vi "836_SetCameraConfiguration.vi"(6 "Vision Fix":bool, 8 "error in (no error)":errorcluster, 9 "Camera Controls":T1, 10 "Initialize":bool, 11 "CameraDevRef":T3={"Camera Address"="USB 0", "CameraStatus"={"status"=FALSE, "code"=0, "source"=""}}) -> (0 "error out":errorcluster, 1 "VideoMode":T2=78 items=["640 x 480 YUY 2 30.00 fps", "640 x 480 YUY 2 20.00 fps", "640 x 480 YUY 2 15.00 fps", "640 x 480 YUY 2 10.00 fps", "640 x 480 YUY 2 7.50 fps", "1280 x 720 YUY 2 10.00 fps", "1280 x 720 YUY 2 7.50 fps", "960 x 544 YUY 2 15.00 fps", "960 x 544 YUY 2 10.00 fps", "960 x 544 YUY 2 7.50 fps", "800 x 448 YUY 2 20.00 fps", "800 x 448 YUY 2 15.00 fps", "800 x 448 YUY 2 10.00 fps", "800 x 448 YUY 2 7.50 fps", "640 x 360 YUY 2 30.00 fps", "640 x 360 YUY 2 20.00 fps", "640 x 360 YUY 2 15.00 fps", "640 x 360 YUY 2 10.00 fps", "640 x 360 YUY 2 7.50 fps", "424 x 240 YUY 2 30.00 fps", "424 x 240 YUY 2 20.00 fps", "424 x 240 YUY 2 15.00 fps", "424 x 240 YUY 2 10.00 fps", "424 x 240 YUY 2 7.50 fps", "352 x 288 YUY 2 30.00 fps", "352 x 288 YUY 2 20.00 fps", "352 x 288 YUY 2 15.00 fps", "352 x 288 YUY 2 10.00 fps", "352 x 288 YUY 2 7.50 fps", "320 x 240 YUY 2 30.00 fps", "320 x 240 YUY 2 20.00 fps", "320 x 240 YUY 2 15.00 fps", "320 x 240 YUY 2 10.00 fps", "320 x 240 YUY 2 7.50 fps", "800 x 600 YUY 2 15.00 fps", "800 x 600 YUY 2 10.00 fps", "800 x 600 YUY 2 7.50 fps", "176 x 144 YUY 2 30.00 fps", "176 x 144 YUY 2 20.00 fps", "176 x 144 YUY 2 15.00 fps", "176 x 144 YUY 2 10.00 fps", "176 x 144 YUY 2 7.50 fps", "160 x 120 YUY 2 30.00 fps", "160 x 120 YUY 2 20.00 fps", "160 x 120 YUY 2 15.00 fps", "160 x 120 YUY 2 10.00 fps", "160 x 120 YUY 2 7.50 fps", "1280 x 800 YUY 2 10.00 fps", "640 x 480 JPEG 30.00 fps", "640 x 480 JPEG 20.00 fps", "640 x 480 JPEG 15.00 fps", "640 x 480 JPEG 10.00 fps", "640 x 480 JPEG 7.50 fps", "1280 x 720 JPEG 30.00 fps", "1280 x 720 JPEG 20.00 fps", "1280 x 720 JPEG 15.00 fps", "1280 x 720 JPEG 10.00 fps", "1280 x 720 JPEG 7.50 fps", "960 x 544 JPEG 30.00 fps", "960 x 544 JPEG 20.00 fps", "960 x 544 JPEG 15.00 fps", "960 x 544 JPEG 10.00 fps", "960 x 544 JPEG 7.50 fps", "800 x 448 JPEG 30.00 fps", "800 x 448 JPEG 20.00 fps", "800 x 448 JPEG 15.00 fps", "800 x 448 JPEG 10.00 fps", "800 x 448 JPEG 7.50 fps", "640 x 360 JPEG 30.00 fps", "640 x 360 JPEG 20.00 fps", "640 x 360 JPEG 15.00 fps", "640 x 360 JPEG 10.00 fps", "640 x 360 JPEG 7.50 fps", "800 x 600 JPEG 30.00 fps", "800 x 600 JPEG 20.00 fps", "800 x 600 JPEG 15.00 fps", "800 x 600 JPEG 10.00 fps", "800 x 600 JPEG 7.50 fps", "416 x 240 JPEG 30.00 fps", "416 x 240 JPEG 20.00 fps", "416 x 240 JPEG 15.00 fps", "416 x 240 JPEG 10.00 fps", "416 x 240 JPEG 7.50 fps", "352 x 288 JPEG 30.00 fps", "352 x 288 JPEG 20.00 fps", "352 x 288 JPEG 15.00 fps", "352 x 288 JPEG 10.00 fps", "352 x 288 JPEG 7.50 fps", "176 x 144 JPEG 30.00 fps", "176 x 144 JPEG 20.00 fps", "176 x 144 JPEG 15.00 fps", "176 x 144 JPEG 10.00 fps", "176 x 144 JPEG 7.50 fps", "320 x 240 JPEG 30.00 fps", "320 x 240 JPEG 20.00 fps", "320 x 240 JPEG 15.00 fps", "320 x 240 JPEG 10.00 fps", "320 x 240 JPEG 7.50 fps", "160 x 120 JPEG 30.00 fps", "160 x 120 JPEG 20.00 fps", "160 x 120 JPEG 15.00 fps", "160 x 120 JPEG 10.00 fps", "160 x 120 JPEG 7.50 fps"], 2 "output cluster":T1, 3 "CameraDevRef 2":T3={"Camera Address"="USB 0", "CameraStatus"={"status"=FALSE, "code"=0, "source"=""}})   [LabVIEW 2015]
uses:
  <vilib>/Rock Robotics/WPI/Camera/WPI_CameraDevRef.ctl
  38 Video Mode.ctl
  <vilib>/userdefined/High Color/IMAQdx.ctl
  <resource>/objmgr/imaqdx.rc
  <vilib>/vision/driver/NI_Vision_Acquisition_Software.lvlib
panel:
  out "error out 2":errorcluster
  in  "VideoModes":T2=81 items=["640 x 480 YUY 2 30.00 fps", "640 x 480 YUY 2 20.00 fps", "640 x 480 YUY 2 15.00 fps", "640 x 480 YUY 2 10.00 fps", "640 x 480 YUY 2 7.50 fps", "1280 x 720 YUY 2 10.00 fps", "1280 x 720 YUY 2 7.50 fps", "960 x 544 YUY 2 15.00 fps", "960 x 544 YUY 2 10.00 fps", "960 x 544 YUY 2 7.50 fps", "800 x 448 YUY 2 20.00 fps", "800 x 448 YUY 2 15.00 fps", "800 x 448 YUY 2 10.00 fps", "800 x 448 YUY 2 7.50 fps", "640 x 360 YUY 2 30.00 fps", "640 x 360 YUY 2 20.00 fps", "640 x 360 YUY 2 15.00 fps", "640 x 360 YUY 2 10.00 fps", "640 x 360 YUY 2 7.50 fps", "424 x 240 YUY 2 30.00 fps", "424 x 240 YUY 2 20.00 fps", "424 x 240 YUY 2 15.00 fps", "424 x 240 YUY 2 10.00 fps", "424 x 240 YUY 2 7.50 fps", "352 x 288 YUY 2 30.00 fps", "352 x 288 YUY 2 20.00 fps", "352 x 288 YUY 2 15.00 fps", "352 x 288 YUY 2 10.00 fps", "352 x 288 YUY 2 7.50 fps", "320 x 240 YUY 2 30.00 fps", "320 x 240 YUY 2 20.00 fps", "320 x 240 YUY 2 15.00 fps", "320 x 240 YUY 2 10.00 fps", "320 x 240 YUY 2 7.50 fps", "800 x 600 YUY 2 15.00 fps", "800 x 600 YUY 2 10.00 fps", "800 x 600 YUY 2 7.50 fps", "176 x 144 YUY 2 30.00 fps", "176 x 144 YUY 2 20.00 fps", "176 x 144 YUY 2 15.00 fps", "176 x 144 YUY 2 10.00 fps", "176 x 144 YUY 2 7.50 fps", "160 x 120 YUY 2 30.00 fps", "160 x 120 YUY 2 20.00 fps", "160 x 120 YUY 2 15.00 fps", "160 x 120 YUY 2 10.00 fps", "160 x 120 YUY 2 7.50 fps", "1280 x 800 YUY 2 10.00 fps", "640 x 480 JPEG 30.00 fps", "640 x 480 JPEG 20.00 fps", "640 x 480 JPEG 15.00 fps", "640 x 480 JPEG 10.00 fps", "640 x 480 JPEG 7.50 fps", "1280 x 720 JPEG 30.00 fps", "1280 x 720 JPEG 20.00 fps", "1280 x 720 JPEG 15.00 fps", "1280 x 720 JPEG 10.00 fps", "1280 x 720 JPEG 7.50 fps", "960 x 544 JPEG 30.00 fps", "960 x 544 JPEG 20.00 fps", "960 x 544 JPEG 15.00 fps", "960 x 544 JPEG 10.00 fps", "960 x 544 JPEG 7.50 fps", "800 x 448 JPEG 30.00 fps", "800 x 448 JPEG 20.00 fps", "800 x 448 JPEG 15.00 fps", "800 x 448 JPEG 10.00 fps", "800 x 448 JPEG 7.50 fps", "640 x 360 JPEG 30.00 fps", "640 x 360 JPEG 20.00 fps", "640 x 360 JPEG 15.00 fps", "640 x 360 JPEG 10.00 fps", "640 x 360 JPEG 7.50 fps", "800 x 600 JPEG 30.00 fps", "800 x 600 JPEG 20.00 fps", "800 x 600 JPEG 15.00 fps", "800 x 600 JPEG 10.00 fps", "800 x 600 JPEG 7.50 fps", "416 x 240 JPEG 30.00 fps", "416 x 240 JPEG 20.00 fps", "416 x 240 JPEG 15.00 fps", "416 x 240 JPEG 10.00 fps", "416 x 240 JPEG 7.50 fps", "352 x 288 JPEG 30.00 fps", "352 x 288 JPEG 20.00 fps", "352 x 288 JPEG 15.00 fps", "352 x 288 JPEG 10.00 fps", "352 x 288 JPEG 7.50 fps", "176 x 144 JPEG 30.00 fps", "176 x 144 JPEG 20.00 fps", "176 x 144 JPEG 15.00 fps", "176 x 144 JPEG 10.00 fps", "176 x 144 JPEG 7.50 fps", "320 x 240 JPEG 30.00 fps", "320 x 240 JPEG 20.00 fps", "320 x 240 JPEG 15.00 fps", "320 x 240 JPEG 10.00 fps", "320 x 240 JPEG 7.50 fps", "160 x 120 JPEG 30.00 fps", "160 x 120 JPEG 20.00 fps", "160 x 120 JPEG 15.00 fps", "160 x 120 JPEG 10.00 fps", "160 x 120 JPEG 7.50 fps"]
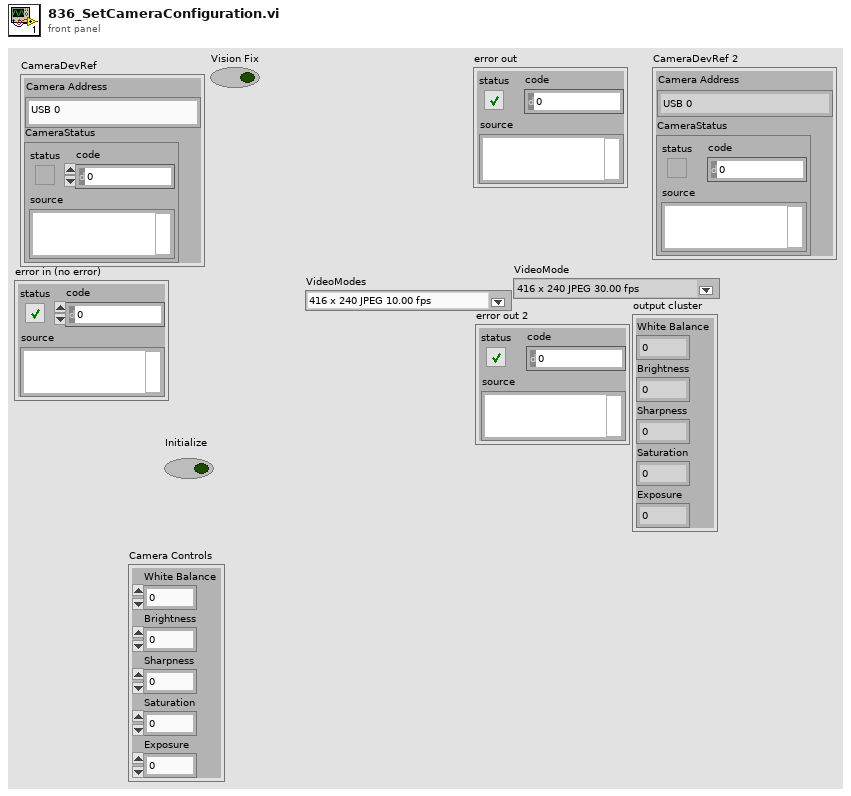
[diagram p1: front panel]
types:
  T1 = cluster{"White Balance":i64, "Brightness":i64, "Sharpness":i64, "Saturation":i64, "Exposure":i64}
  T2 = typedef "38 Video Mode.ctl" = u32
  T3 = typedef "WPI_CameraDevRef.ctl" = cluster{"Camera Address":string, "CameraStatus":errorcluster}
  T4 = typedef "IMAQdx.ctl" = refnum<k21>
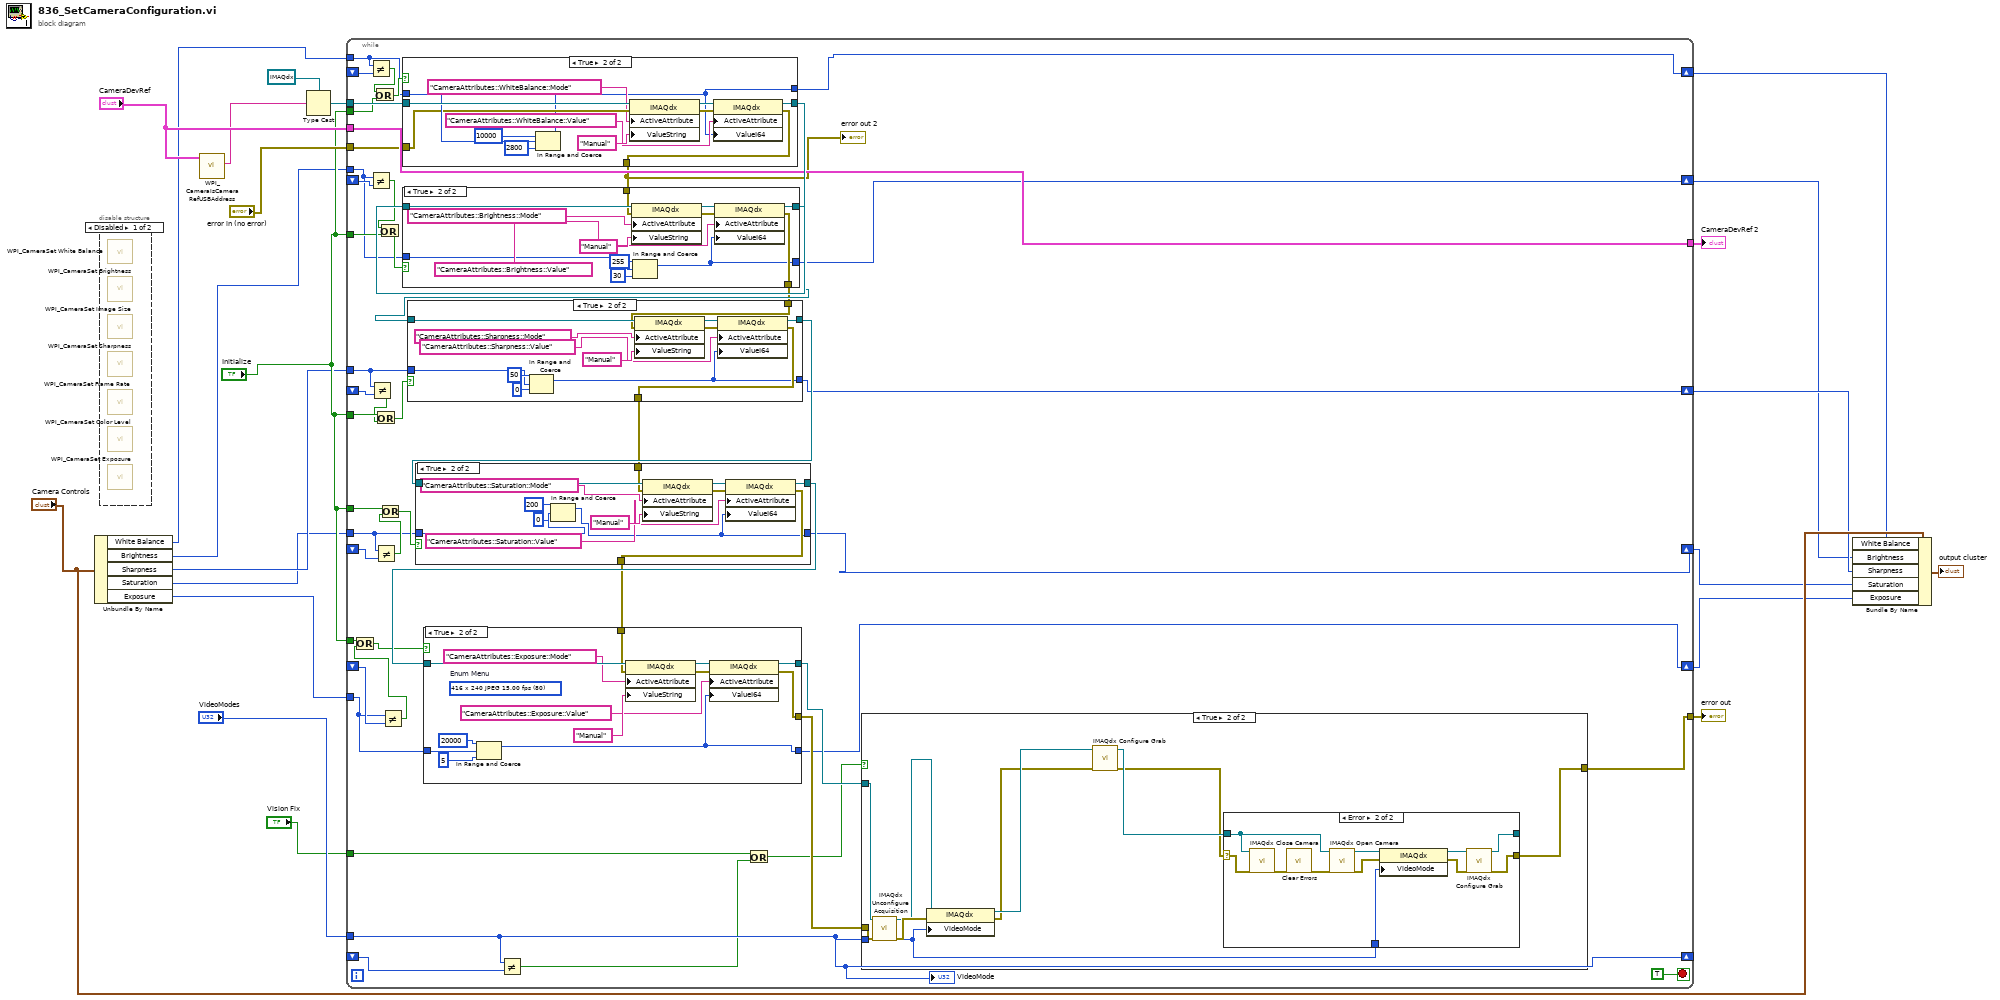
[diagram p0: block diagram]
diagram:
  n1 = Unbundle By Name("Camera Controls") -> ("White Balance"=w13:i64, "Brightness"=w12:i64, "Sharpness"=w11:i64, "Saturation"=w10:i64, "Exposure"=w9:i64)
  n2 = disable-structure shown="Disabled" {
    frame Disabled {
      n3 = call <vilib>:"WPI_CameraSet White Balance.vi"() -> ()  [unwired: 10 in, 2 out]
      n4 = call <vilib>:"WPI_CameraSet Brightness.vi"() -> ()  [unwired: 10 in, 2 out]
      n5 = call <vilib>:"WPI_CameraSet Image Size.vi"() -> ()  [unwired: 10 in, 2 out]
      n6 = call <vilib>:"WPI_CameraSet Sharpness.vi"() -> ()  [unwired: 10 in, 2 out]
      n7 = call <vilib>:"WPI_CameraSet Frame Rate.vi"() -> ()  [unwired: 10 in, 2 out]
      n8 = call <vilib>:"WPI_CameraSet Color Level.vi"() -> ()  [unwired: 10 in, 2 out]
      n9 = call <vilib>:"WPI_CameraSet Exposure.vi"() -> ()  [unwired: 10 in, 2 out]
    }
    frame Enabled {
    }
  }
  n10 = call <vilib>:"WPI_CameraIsCameraRefUSBAddress.vi"("CameraDevRef"="CameraDevRef") -> ("Camera Address Out"=w15:string)  [unwired: 7 in, 3 out]
  n11 = Type Cast(type=T4 refnum ("IMAQdx Session"), x=w15) -> (*(type *) &x=w22:T4)
  n12 = while {
    tunnel: w13 -> [w31]
    tunnel: w22 -> [w72]
    shift-right: [w30] -> w3
    shift-left: _ -> [w71]
    shift-right: [w32] -> w4
    shift-left: _ -> [w69]
    tunnel: w12 -> [w33]
    tunnel: w11 -> [w66]
    shift-right: [w34] -> w5
    shift-left: _ -> [w67]
    tunnel: "CameraDevRef" -> [w63]
    tunnel: [w63] -> w20
    tunnel: w10 -> [w29]
    tunnel: w9 -> [w27]
    shift-right: [w28] -> w6
    shift-left: _ -> [w61]
    shift-right: [w26] -> w7
    shift-left: _ -> [w60]
    tunnel: "VideoModes" -> [w50]
    tunnel: [w52] -> w18
    tunnel: "error in (no error)" -> [w56]
    shift-right: [w50] -> _
    shift-left: _ -> [w51]
    tunnel: "Initialize" -> [w48]
    tunnel: "Initialize" -> [w45]
    tunnel: "Initialize" -> [w42]
    tunnel: "Initialize" -> [w38]
    tunnel: "Initialize" -> [w35]
    tunnel: "Vision Fix" -> [w23]
    stop <- TRUE stop-if-true
    n13 = Not Equal?(x=w31, y=w71) -> (x != y?=w49:bool)
    n14 = Not Equal?(x=w33, y=w69) -> (x != y?=w46:bool)
    n15 = Not Equal?(x=w66, y=w67) -> (x != y?=w41:bool)
    n16 = Or(x=w49, y=w48) -> (x .or. y?=w47:bool)
    n17 = Or(x=w42, y=w41) -> (x .or. y?=w43:bool)
    n18 = Not Equal?(x=w29, y=w61) -> (x != y?=w39:bool)
    n19 = Or(x=w46, y=w45) -> (x .or. y?=w44:bool)
    n20 = Or(x=w38, y=w39) -> (x .or. y?=w40:bool)
    n21 = Not Equal?(x=w27, y=w60) -> (x != y?=w36:bool)
    n22 = Or(x=w35, y=w36) -> (x .or. y?=w37:bool)
    n23 = case shown="True" w47 {
      tunnel: w72 -> [w163 w175]
      tunnel: w31 -> [w161 w170]
      tunnel: [w163 w173] -> w70
      tunnel: [w162 w169] -> w55
      tunnel: w56 -> [w162 w167]
      tunnel: [w161 w164] -> w30
      frame False {
      }
      frame True {
        n24 = In Range and Coerce(upper limit=i64 10000, x=w170, lower limit=i64 2800) -> (coerced(x)=w164:i64)  [unwired: 1 out]
        n25 = property class="IMAQdx"(reference=w175, error in=w167, "ActiveAttribute"="CameraAttributes::WhiteBalance::Mode", "ValueString"="Manual") -> (reference out=w176:T4, error out=w168:errorcluster)
        n26 = property class="IMAQdx"(reference=w176, error in=w168, "ActiveAttribute"="CameraAttributes::WhiteBalance::Value", "ValueI64"=w164) -> (reference out=w173:T4, error out=w169:errorcluster)
      }
    }
    "error out 2" <- w55
    n27 = case shown="True" w44 {
      tunnel: w70 -> [w147 w159]
      tunnel: [w147 w157] -> w68
      tunnel: w33 -> [w145 w153]
      tunnel: [w146 w152] -> w57
      tunnel: w55 -> [w146 w150]
      tunnel: [w145 w148] -> w32
      frame False {
      }
      frame True {
        n28 = property class="IMAQdx"(reference=w159, error in=w150, "ActiveAttribute"="CameraAttributes::Brightness::Mode", "ValueString"="Manual") -> (reference out=w160:T4, error out=w151:errorcluster)
        n29 = In Range and Coerce(upper limit=i64 255, x=w153, lower limit=i64 30) -> (coerced(x)=w148:i64)  [unwired: 1 out]
        n30 = property class="IMAQdx"(reference=w160, error in=w151, "ActiveAttribute"="CameraAttributes::Brightness::Value", "ValueI64"=w148) -> (reference out=w157:T4, error out=w152:errorcluster)
      }
    }
    n31 = case shown="True" w43 {
      tunnel: w68 -> [w131 w143]
      tunnel: [w131 w141] -> w65
      tunnel: w66 -> [w129 w137]
      tunnel: [w130 w136] -> w58
      tunnel: w57 -> [w130 w134]
      tunnel: [w129 w132] -> w34
      frame False {
      }
      frame True {
        n32 = In Range and Coerce(upper limit=i64 50, x=w137, lower limit=i64 0) -> (coerced(x)=w132:i64)  [unwired: 1 out]
        n33 = property class="IMAQdx"(reference=w143, error in=w134, "ActiveAttribute"="CameraAttributes::Sharpness::Mode", "ValueString"="Manual") -> (reference out=w144:T4, error out=w135:errorcluster)
        n34 = property class="IMAQdx"(reference=w144, error in=w135, "ActiveAttribute"="CameraAttributes::Sharpness::Value", "ValueI64"=w132) -> (reference out=w141:T4, error out=w136:errorcluster)
      }
    }
    n35 = case shown="True" w40 {
      tunnel: w65 -> [w115 w127]
      tunnel: [w115 w125] -> w64
      tunnel: w29 -> [w113 w123]
      tunnel: [w114 w120] -> w59
      tunnel: w58 -> [w114 w118]
      tunnel: [w113 w116] -> w28
      frame False {
      }
      frame True {
        n36 = In Range and Coerce(upper limit=i64 200, x=w123, lower limit=i64 0) -> (coerced(x)=w116:i64)  [unwired: 1 out]
        n37 = property class="IMAQdx"(reference=w127, error in=w118, "ActiveAttribute"="CameraAttributes::Saturation::Mode", "ValueString"="Manual") -> (reference out=w128:T4, error out=w119:errorcluster)
        n38 = property class="IMAQdx"(reference=w128, error in=w119, "ActiveAttribute"="CameraAttributes::Saturation::Value", "ValueI64"=w116) -> (reference out=w125:T4, error out=w120:errorcluster)
      }
    }
    n39 = case shown="True" w37 {
      tunnel: w64 -> [w99 w111]
      tunnel: [w99 w109] -> w53
      tunnel: w27 -> [w97 w107]
      tunnel: [w98 w104] -> w54
      tunnel: w59 -> [w98 w102]
      tunnel: [w97 w100] -> w26
      frame False {
      }
      frame True {
        (unwired) T2 80 items=["640 x 480 YUY 2 30.00 fps", "640 x 480 YUY 2 20.00 fps", "640 x 480 YUY 2 15.00 fps", "640 x 480 YUY 2 10.00 fps", "640 x 480 YUY 2 7.50 fps", "1280 x 720 YUY 2 10.00 fps", "1280 x 720 YUY 2 7.50 fps", "960 x 544 YUY 2 15.00 fps", "960 x 544 YUY 2 10.00 fps", "960 x 544 YUY 2 7.50 fps", "800 x 448 YUY 2 20.00 fps", "800 x 448 YUY 2 15.00 fps", "800 x 448 YUY 2 10.00 fps", "800 x 448 YUY 2 7.50 fps", "640 x 360 YUY 2 30.00 fps", "640 x 360 YUY 2 20.00 fps", "640 x 360 YUY 2 15.00 fps", "640 x 360 YUY 2 10.00 fps", "640 x 360 YUY 2 7.50 fps", "424 x 240 YUY 2 30.00 fps", "424 x 240 YUY 2 20.00 fps", "424 x 240 YUY 2 15.00 fps", "424 x 240 YUY 2 10.00 fps", "424 x 240 YUY 2 7.50 fps", "352 x 288 YUY 2 30.00 fps", "352 x 288 YUY 2 20.00 fps", "352 x 288 YUY 2 15.00 fps", "352 x 288 YUY 2 10.00 fps", "352 x 288 YUY 2 7.50 fps", "320 x 240 YUY 2 30.00 fps", "320 x 240 YUY 2 20.00 fps", "320 x 240 YUY 2 15.00 fps", "320 x 240 YUY 2 10.00 fps", "320 x 240 YUY 2 7.50 fps", "800 x 600 YUY 2 15.00 fps", "800 x 600 YUY 2 10.00 fps", "800 x 600 YUY 2 7.50 fps", "176 x 144 YUY 2 30.00 fps", "176 x 144 YUY 2 20.00 fps", "176 x 144 YUY 2 15.00 fps", "176 x 144 YUY 2 10.00 fps", "176 x 144 YUY 2 7.50 fps", "160 x 120 YUY 2 30.00 fps", "160 x 120 YUY 2 20.00 fps", "160 x 120 YUY 2 15.00 fps", "160 x 120 YUY 2 10.00 fps", "160 x 120 YUY 2 7.50 fps", "1280 x 800 YUY 2 10.00 fps", "640 x 480 JPEG 30.00 fps", "640 x 480 JPEG 20.00 fps", "640 x 480 JPEG 15.00 fps", "640 x 480 JPEG 10.00 fps", "640 x 480 JPEG 7.50 fps", "1280 x 720 JPEG 30.00 fps", "1280 x 720 JPEG 20.00 fps", "1280 x 720 JPEG 15.00 fps", "1280 x 720 JPEG 10.00 fps", "1280 x 720 JPEG 7.50 fps", "960 x 544 JPEG 30.00 fps", "960 x 544 JPEG 20.00 fps", "960 x 544 JPEG 15.00 fps", "960 x 544 JPEG 10.00 fps", "960 x 544 JPEG 7.50 fps", "800 x 448 JPEG 30.00 fps", "800 x 448 JPEG 20.00 fps", "800 x 448 JPEG 15.00 fps", "800 x 448 JPEG 10.00 fps", "800 x 448 JPEG 7.50 fps", "640 x 360 JPEG 30.00 fps", "640 x 360 JPEG 20.00 fps", "640 x 360 JPEG 15.00 fps", "640 x 360 JPEG 10.00 fps", "640 x 360 JPEG 7.50 fps", "800 x 600 JPEG 30.00 fps", "800 x 600 JPEG 20.00 fps", "800 x 600 JPEG 15.00 fps", "800 x 600 JPEG 10.00 fps", "800 x 600 JPEG 7.50 fps", "416 x 240 JPEG 30.00 fps", "416 x 240 JPEG 20.00 fps", "416 x 240 JPEG 15.00 fps", "416 x 240 JPEG 10.00 fps", "416 x 240 JPEG 7.50 fps", "352 x 288 JPEG 30.00 fps", "352 x 288 JPEG 20.00 fps", "352 x 288 JPEG 15.00 fps", "352 x 288 JPEG 10.00 fps", "352 x 288 JPEG 7.50 fps", "176 x 144 JPEG 30.00 fps", "176 x 144 JPEG 20.00 fps", "176 x 144 JPEG 15.00 fps", "176 x 144 JPEG 10.00 fps", "176 x 144 JPEG 7.50 fps", "320 x 240 JPEG 30.00 fps", "320 x 240 JPEG 20.00 fps", "320 x 240 JPEG 15.00 fps", "320 x 240 JPEG 10.00 fps", "320 x 240 JPEG 7.50 fps", "160 x 120 JPEG 30.00 fps", "160 x 120 JPEG 20.00 fps", "160 x 120 JPEG 15.00 fps", "160 x 120 JPEG 10.00 fps", "160 x 120 JPEG 7.50 fps"]  # Enum Menu
        n40 = In Range and Coerce(upper limit=i64 20000, x=w107, lower limit=i64 5) -> (coerced(x)=w100:i64)  [unwired: 1 out]
        n41 = property class="IMAQdx"(reference=w111, error in=w102, "ActiveAttribute"="CameraAttributes::Exposure::Mode", "ValueString"="Manual") -> (reference out=w112:T4, error out=w103:errorcluster)
        n42 = property class="IMAQdx"(reference=w112, error in=w103, "ActiveAttribute"="CameraAttributes::Exposure::Value", "ValueI64"=w100) -> (reference out=w109:T4, error out=w104:errorcluster)
      }
    }
    n43 = Not Equal?(x=w50, y=w51) -> (x != y?=w25:bool)
    n44 = Or(x=w23, y=w25) -> (x .or. y?=w24:bool)
    n45 = case shown="True" w24 {
      tunnel: w50 -> [_ w76]
      tunnel: w54 -> [w73 w83]
      tunnel: w53 -> [_ w82]
      tunnel: [w73 w74] -> w52
      frame False {
      }
      frame True {
        n46 = call <vilib>:"IMAQdx Unconfigure Acquisition.vi"("error in"=w83, "Session In"=w82) -> ("error out"=w81:errorcluster, "Session Out"=w80:T4)  [unwired: 8 in]
        n47 = property class="IMAQdx"(reference=w80, error in=w81, "VideoMode"=w76) -> (reference out=w79:T4, error out=w78:errorcluster)
        n48 = call <vilib>:"IMAQdx Configure Grab.vi"("error in"=w78, "Session In"=w79) -> ("error out"=w75:errorcluster, "Session Out"=w77:T4)  [unwired: 8 in]
        n49 = case shown="Error" w75 {
          selector: w75 -> [w85 w87]
          tunnel: [w85 w93] -> w74
          tunnel: w77 -> [w84 w88]
          tunnel: [w84 w94] -> _
          tunnel: w76 -> [_ w86]
          frame No Error {
          }
          frame Error {
            n50 = call <vilib>:"IMAQdx Close Camera.vi"("error in"=w87, "Session In"=w88) -> ("error out"=w96:errorcluster)  [unwired: 9 in]
            n51 = call <vilib>:"Clear Errors.vi"("error in (no error)"=w96) -> ("error out"=w95:errorcluster)  [unwired: 5 in, 1 out]
            n52 = call <vilib>:"IMAQdx Open Camera.vi"("error in"=w95, "Session In"=w88) -> ("error out"=w90:errorcluster, "Session Out"=w92:T4)  [unwired: 8 in]
            n53 = property class="IMAQdx"(reference=w92, error in=w90, "VideoMode"=w86) -> (reference out=w91:T4, error out=w89:errorcluster)
            n54 = call <vilib>:"IMAQdx Configure Grab.vi"("error in"=w89, "Session In"=w91) -> ("error out"=w93:errorcluster, "Session Out"=w94:T4)  [unwired: 8 in]
          }
        }
      }
    }
    "VideoMode" <- w50
  }
  "CameraDevRef 2" <- w20
  "error out" <- w18
  n55 = Bundle By Name(cluster="Camera Controls", "White Balance"=w3, "Brightness"=w4, "Sharpness"=w5, "Saturation"=w6, "Exposure"=w7) -> (→"output cluster":T1)
